vi "Create Class.vi"(8 "error in (no error)":errorcluster, 11 "Message Maker in":refnum<class "Message Scripter.lvclass">) -> (0 "error out":errorcluster, 3 "Message Maker out":refnum<class "Message Scripter.lvclass">)   [LabVIEW 2020, in "Message Maker.lvlib" / "Message Scripter.lvclass"]
uses:
  Message Scripter.lvclass
  Message Maker.lvlib
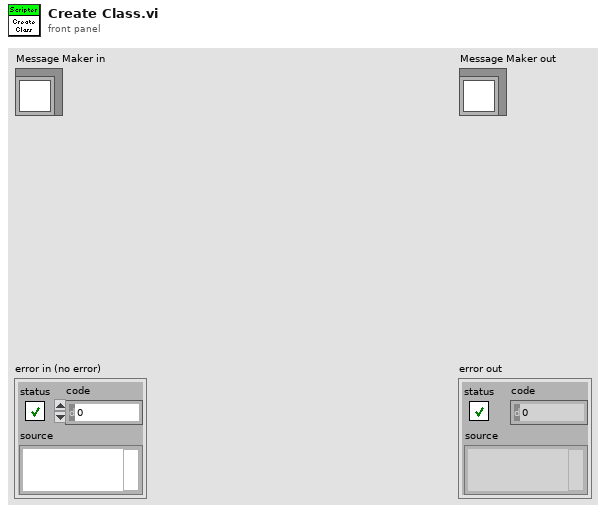
[diagram p1: front panel]
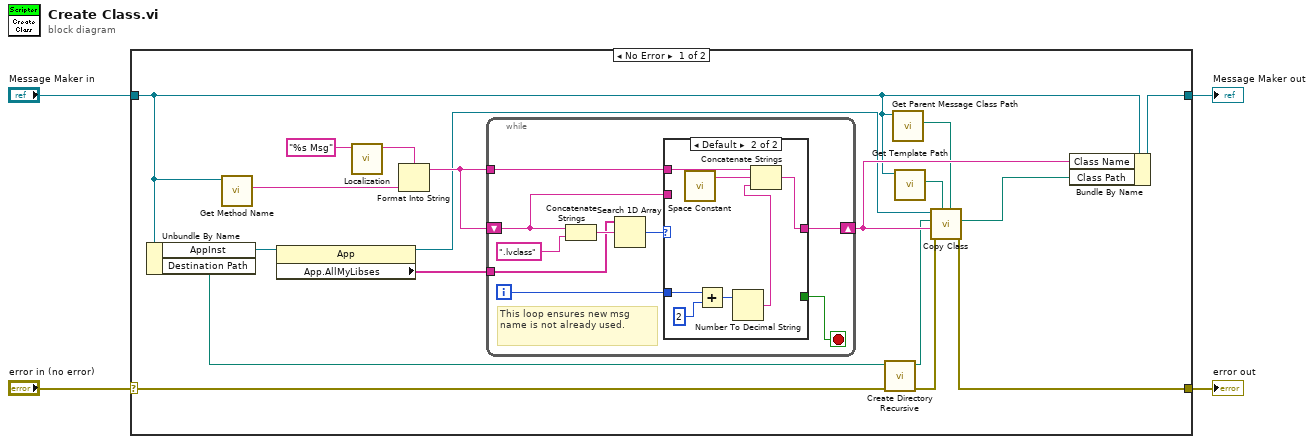
[diagram p0: block diagram]
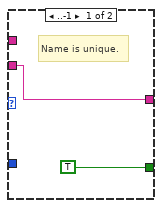
[diagram p2: hidden frame]
diagram:
  n1 = case shown="No Error" "error in (no error)" {
    selector: "error in (no error)" -> [w9 w42]
    tunnel: [w11 w42] -> w3
    tunnel: [w13 w41] -> w1
    tunnel: "Message Maker in" -> [w5 w41]
    frame No Error {
      n2 = Unbundle By Name(w5) -> ("AppInst"=w18:refnum<vi>, "Destination Path"=w10:path)
      n3 = call-dynamic "Get Method Name.vi"("Message Maker in"=w5) -> ("Method Name"=w6:string)  [unwired: 10 in]
      n4 = property class="App"(reference=w18) -> (reference out=w15:refnum<vi>, "App.AllMyLibses"=w20:string[])  [unwired: 1 in, 1 out]
      n5 = call "Localization.vi"("Unlocalized"="%s Msg" ("Name of new Message Class (without .lvclass file extension)")) -> ("Localized"=w22:string)  [unwired: 10 in]
      n6 = Format Into String(format string=w22, w6) -> (resulting string=w19:string)  [unwired: 2 in, 1 out]
      n7 = while {
        tunnel: w19 -> [w27]
        shift-right: [w24] -> w16
        shift-left: w19 -> [w26]
        tunnel: w20 -> [w29]
        i -> [w25]
        stop <- w23 stop-if-true
        # "This loop ensures new msg name is not already used."
        n8 = Concatenate Strings(w26, ".lvclass" ("string")) -> (w30:string)
        n9 = Search 1D Array(1D array=w29, element=w30) -> (index of element=w28:i32)  [unwired: 1 in]
        n10 = case shown="Default" w28 {
          tunnel: w27 -> [_ w40]
          tunnel: w26 -> [w33 _]
          tunnel: w25 -> [_ w38]
          tunnel: [w33 w34] -> w24
          tunnel: [TRUE _] -> w23
          frame ..-1 {
            # "Name is unique."
          }
          frame Default {
            n11 = call <vilib>:"Space Constant.vi"() -> ("String"=w39:string)
            n12 = Add(x=w38, y=2) -> (x+y=w36:i32)
            n13 = Number To Decimal String(number=w36) -> (decimal integer string=w35:string)  [unwired: 1 in]
            n14 = Concatenate Strings(w40, w39, w35) -> (w34:string)
          }
        }
      }
      n15 = call <vilib>:"Create Directory Recursive.vi"("error in (no error)"=w9, "directory"=w10) -> ("error out"=w7:errorcluster, "directory copy"=w8:path)  [unwired: 3 in, 1 out]
      n16 = call-dynamic "Get Parent Message Class Path.vi"("Message Scripter in"=w5) -> ("Parent Message"=w14:path)  [unwired: 9 in, 1 out]
      n17 = call-dynamic "Get Template Path.vi"("Message Maker in"=w5) -> ("Template Path"=w17:path)  [unwired: 10 in]
      n18 = call "Copy Class.vi"("Parent Class Path"=w14, "Template Path"=w17, "error in (no error)"=w7, "Class Name"=w16, "Destination Directory"=w8, "AppInst"=w15) -> ("error out"=w11:errorcluster, "New Class Path"=w12:path)  [unwired: 4 in]
      n19 = Bundle By Name(cluster=w5, "Class Name"=w16, "Class Path"=w12) -> (w13:refnum<class "Message Scripter.lvclass">)
    }
    frame Error {
    }
  }
  "error out" <- w3
  "Message Maker out" <- w1
